vi "VeristandStop.vi"(8 "error in (no error)":errorcluster, 10 "CloseApp?":bool) -> (0 "error out":errorcluster)   [LabVIEW 2015, in "MiscHelperVIs.lvlib"]
uses:
  MiscHelperVIs.lvlib
  <vilib>/NI Veristand/Execution/Project/NI_VS Project ExecutionAPI.lvlib
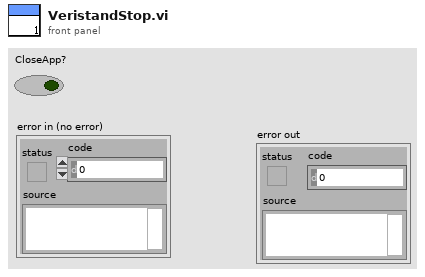
[diagram p1: front panel]
types:
  T1 = typedef "MiscHelperVIs.lvlib/VeriStand dotNet References.ctl" = cluster{"Project Ref":refnum<k24>, "Workspace Manager Ref":refnum<k24>, "Model Manager Ref":refnum<k24>, "Channel Fault Manager Ref":refnum<k24>}
  T2 = typedef "NI_VS Project ExecutionAPI.lvlib/Project Ref.ctl" = refnum<k24>
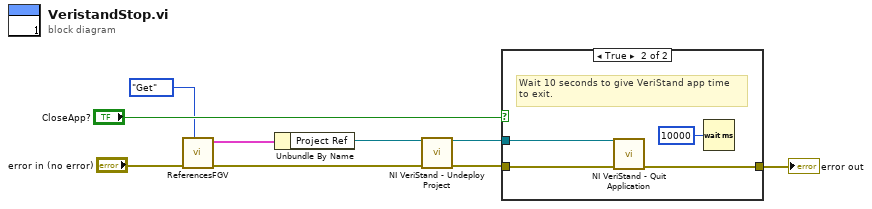
[diagram p0: block diagram]
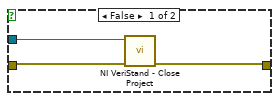
[diagram p2: hidden frame]
diagram:
  n1 = call "ReferencesFGV.vi"("Get/Set"=enum16{"Get", "Set"}."Get", "error in (no error)"="error in (no error)") -> ("error out"=w5:errorcluster, "VeriStand dotNET Refs out"=w2:T1)  [unwired: 8 in]
  n2 = Unbundle By Name(w2) -> ("Project Ref"=w1:refnum<k24>)
  n3 = call <vilib>:"NI VeriStand - Undeploy Project.vi"("error in (no error)"=w5, "Project Ref in"=w1) -> ("error out"=w7:errorcluster, "Project Ref out"=w6:T2)  [unwired: 8 in]
  n4 = case shown="True" "CloseApp?" {
    tunnel: w6 -> [w12 w16]
    tunnel: w7 -> [w11 w15]
    tunnel: [w10 w14] -> w8
    frame False {
      n5 = call <vilib>:"NI VeriStand - Close Project.vi"("error in (no error)"=w11, "Project Ref in"=w12) -> ("error out"=w10:errorcluster)  [unwired: 8 in, 1 out]
    }
    frame True {
      # "Wait 10 seconds to give VeriStand app time\nto exit."
      n6 = call <vilib>:"NI VeriStand - Quit Application.vi"("error in (no error)"=w15, "Project Ref in"=w16) -> ("error out"=w14:errorcluster)  [unwired: 8 in, 1 out]
      n7 = Wait (ms)(milliseconds to wait=u32 10000) -> ()  [unwired: 1 out]
    }
  }
  "error out" <- w8
